vi "Get_Characters_from_string.vi"(2 "Show Dialog?":bool, 3 "Input string":string, 4 "Variable name":string) -> (0 "Status":enum16{"Char in string", "Char not in string"}(ring), 1 "Value":string)   [LabVIEW 2015]
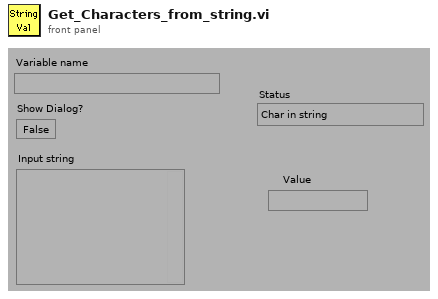
[diagram p1: front panel]
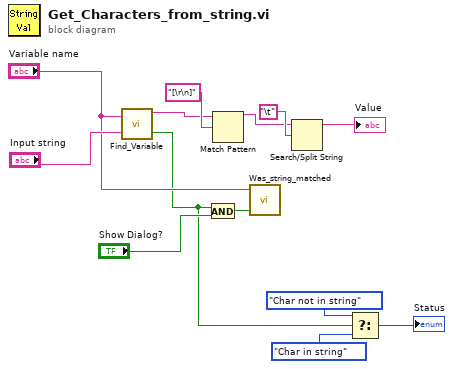
[diagram p0: block diagram]
diagram:
  n1 = call "Find_Variable.vi"("Input string"="Input string", "Variable name"="Variable name") -> ("No Match?"=w2:bool, "After  Matched string"=w9:string)
  n2 = And(x=w2, y="Show Dialog?") -> (x .and. y?=w6:bool)
  n3 = Match Pattern(string=w9, regular expression="[\r\n]") -> (before substring=w8:string)  [unwired: 4 out]
  n4 = call "Was_string_matched.vi"("Match Error"=w6, "Variable name"="Variable name") -> ()  [unwired: 1 in]
  n5 = Search/Split String(string=w8, search string/char (-)="\t") -> (substring before match=→"Value":string)  [unwired: 3 out]
  n6 = Select(t=enum16{"Char in string", "Char not in string"}."Char not in string", s=w2, f=enum16{"Char in string", "Char not in string"}."Char in string") -> (s? t:f=→"Status":enum16{"Char in string", "Char not in string"})
